vi "CRYASIO Play Buffer Stimulus.vi"(0 "Data Array":sgl[](array[numeric]), 1 "Buffer Index":u32, 2 "Buffer Amount":u32, 3 "Limit":u32) -> (9 "Buffer Index Out":u32, 10 "Buffer Amount Out":u32)   [LabVIEW 2013]
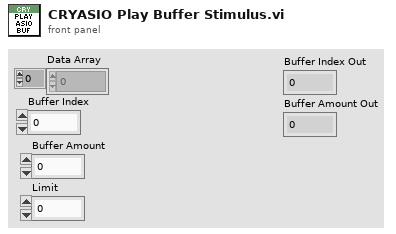
[diagram p1: front panel]
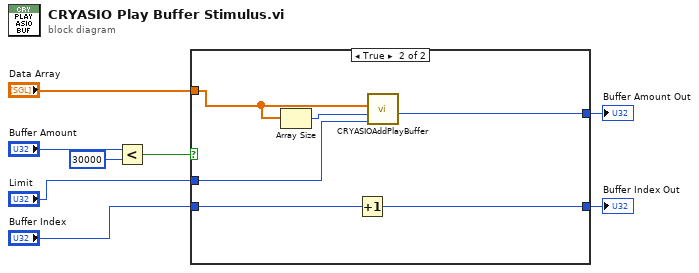
[diagram p0: block diagram]
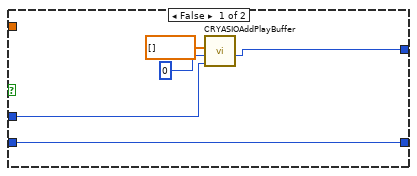
[diagram p2: hidden frame]
diagram:
  n1 = Less?(x="Buffer Amount", y=u32 30000) -> (x < y?=w6:bool)
  n2 = case shown="True" w6 {
    tunnel: "Data Array" -> [_ w17]
    tunnel: "Buffer Index" -> [w13 w19]
    tunnel: [w13 w18] -> w4
    tunnel: "Limit" -> [w10 w15]
    tunnel: [w9 w14] -> w2
    frame False {
      n3 = call "CRYASIOAddPlayBuffer.vi"("Limit"=w10, "Data Length"=0, "pData"=sgl[] []) -> ("Buffer Amount"=w9:i32)  [unwired: 5 in, 2 out]
    }
    frame True {
      n4 = Array Size(array=w17) -> (size(s)=w16:i32)
      n5 = Increment(x=w19) -> (x+1=w18:u32)
      n6 = call "CRYASIOAddPlayBuffer.vi"("Limit"=w15, "Data Length"=w16, "pData"=w17) -> ("Buffer Amount"=w14:i32)  [unwired: 5 in, 2 out]
    }
  }
  "Buffer Index Out" <- w4
  "Buffer Amount Out" <- w2
